vi "CF,BW to Fmin,Fmax.vi"(8 "BW":dbl, 10 "CF":dbl) -> (0 "Fmax":dbl, 2 "Fmin":dbl)   [LabVIEW 2020]
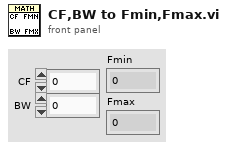
[diagram p1: front panel]
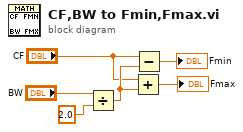
[diagram p0: block diagram]
diagram:
  n1 = Divide(x="BW", y=2.0) -> (x/y=w5:dbl)
  n2 = Add(x="CF", y=w5) -> (x+y=→"Fmax":dbl)
  n3 = Subtract(x="CF", y=w5) -> (x-y=→"Fmin":dbl)
